vi "Inficon - Run process.vi"(8 "Error In":errorcluster, 10 "Run process":bool, 11 "COM port in":refnum<visa-resource-name>) -> (0 "Error Out":errorcluster, 3 "COM port out":refnum<visa-resource-name>)   [LabVIEW 2014]
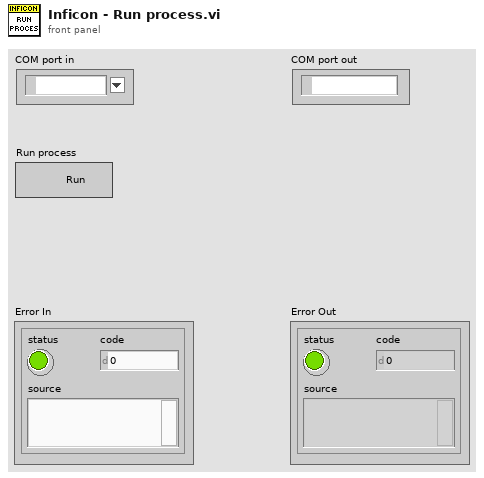
[diagram p1: front panel]
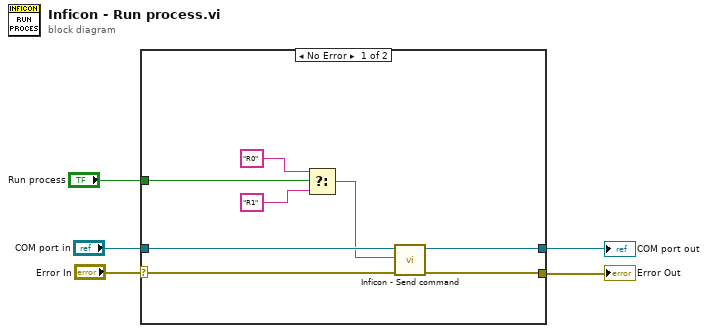
[diagram p0: block diagram]
diagram:
  n1 = case shown="No Error" "Error In" {
    selector: "Error In" -> [w13 w15]
    tunnel: [w12 w15] -> w4
    tunnel: "COM port in" -> [w11 w14]
    tunnel: [w10 w14] -> w2
    tunnel: "Run process" -> [w9 _]
    frame No Error {
      n2 = Select(t="R0", s=w9, f="R1") -> (s? t:f=w7:string)
      n3 = call "Inficon - Send command.vi"("Error In"=w13, "Command"=w7, "COM in"=w11) -> ("Error Out"=w12:errorcluster, "COM out"=w10:refnum<visa-resource-name>)  [unwired: 6 in, 1 out]
    }
    frame Error {
    }
  }
  "Error Out" <- w4
  "COM port out" <- w2
